vi "Coord window-Coord list key focus.vi"(8 "error in (no error)":errorcluster) -> (0 "error out":errorcluster)   [LabVIEW 2020]
uses:
  Globals/Coord window-Globals.vi
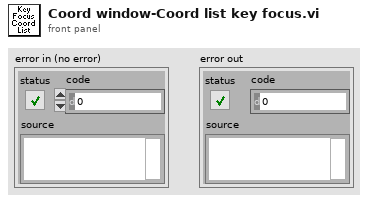
[diagram p1: front panel]
types:
  T1 = typedef "Coordinate list window refs.ctl" = cluster{"Window Name (i.e. Key)":string, "menu reference":refnum<k9>, "VI's reference":refnum<vi>, "Pane 1":refnum<vi>, "Pane 2":refnum<vi>, "Coord Listbox":refnum<vi>, "File name":refnum<vi>, "Picture Map":refnum<vi>, "Stage XYZ Position ind.":refnum<vi>}
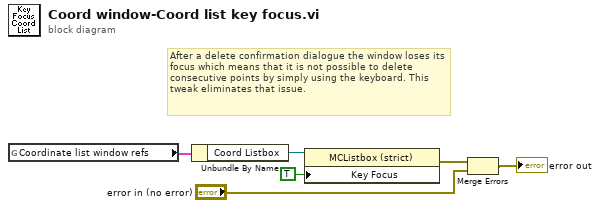
[diagram p0: block diagram]
diagram:
  # "After a delete confirmation dialogue the window loses its focus which means that it is not possible to delete consecutive points by simply using the keyboard. This tweak eliminates that issue."
  n1 = global read "Coord window-Globals.vi" "Coordinate list window refs"() -> (w5:T1)
  n2 = Unbundle By Name(w5) -> ("Coord Listbox"=w6:refnum<vi>)
  n3 = property on="Property Node" class="MCListbox (strict)"(reference=w6, "Key Focus"=TRUE) -> (error out=w3:errorcluster)  [unwired: 1 in, 1 out]
  n4 = Merge Errors(w3, "error in (no error)") -> (→"error out":errorcluster)
